vi "Solution part 2.vi"() -> ()   [LabVIEW 2020]
panel:
  out "Loop results":u64[](array[numeric])
  out "Total result":u64
  in  "data?":bool
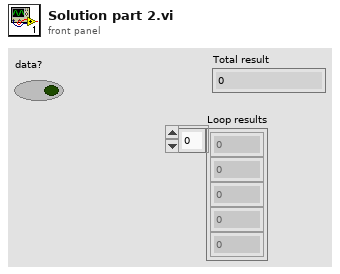
[diagram p1: front panel]
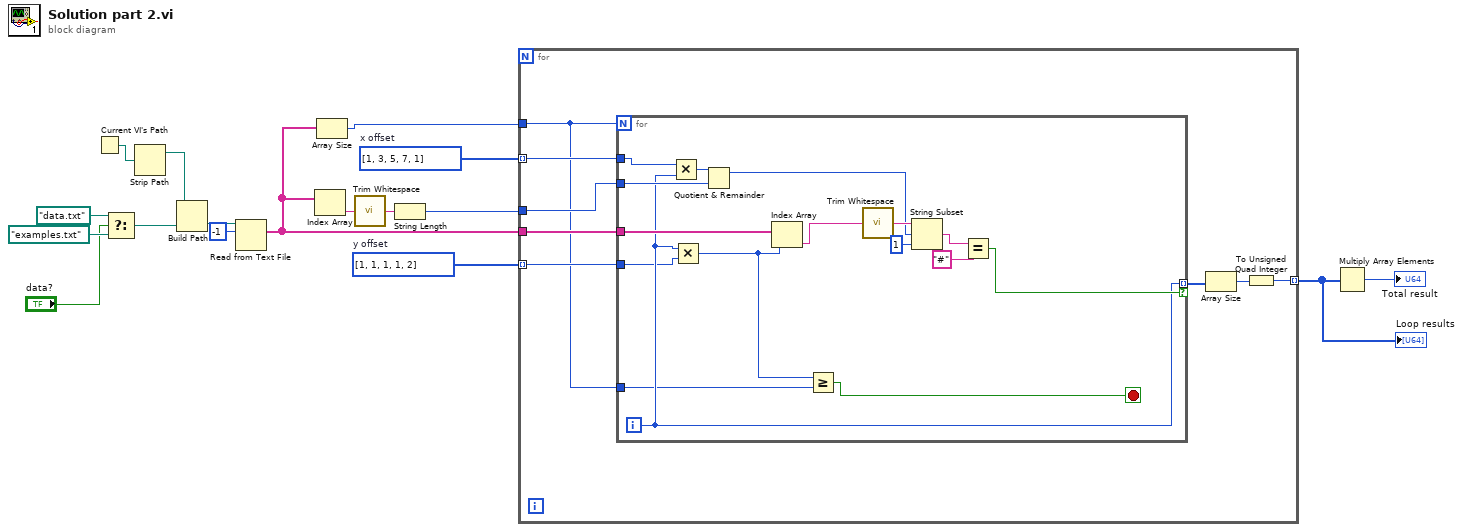
[diagram p0: block diagram]
diagram:
  w1 = i32[] [1, 3, 5, 7, 1]  # x offset
  w2 = i32[] [1, 1, 1, 1, 2]  # y offset
  n1 = Current VI's Path() -> (path=w13:path)
  n2 = Select(t=path "data.txt", s="data?", f=path "examples.txt") -> (s? t:f=w14:path)
  n3 = Strip Path(path=w13) -> (stripped path=w12:path)  [unwired: 1 out]
  n4 = Build Path(base path=w12, name or relative path=w14) -> (appended path=w11:path)
  n5 = Read from Text File(file (use dialog)=w11, count=-1) -> (text=w6:string[])  [unwired: 2 in, 3 out]
  n6 = Index Array(array=w6) -> (element=w9:string)  [unwired: 1 in]
  n7 = Array Size(array=w6) -> (size(s)=w5:i32)
  n8 = call <vilib>:"Trim Whitespace.vi"("string"=w9) -> ("trimmed string"=w7:string)  [unwired: 1 in]
  n9 = String Length(string=w7) -> (length=w8:i32)
  n10 = for {
    tunnel: [w18] -> w4 mode=indexing
    tunnel: w8 -> [w23]
    tunnel: w6 -> [w22]
    tunnel: w5 -> [w19]
    tunnel: w2 -> [w21] mode=indexing
    tunnel: w1 -> [w20] mode=indexing
    n11 = for {
      N: w19 -> [_]
      tunnel: w22 -> [w32]
      tunnel: [w31] -> w25 mode=indexing if=w37
      tunnel: w23 -> [w41]
      tunnel: w20 -> [w35]
      tunnel: w21 -> [w30]
      tunnel: w19 -> [w28]
      i -> [w31]
      stop <- w26 stop-if-true
      n12 = Multiply(x=w35, y=w31) -> (x*y=w34:i32)
      n13 = Multiply(x=w31, y=w30) -> (x*y=w27:i32)
      n14 = Quotient & Remainder(x=w34, y=w41) -> (x-y*floor(x/y)=w33:i32)  [unwired: 1 out]
      n15 = Index Array(array=w32, index=w27) -> (element=w29:string)
      n16 = Greater Or Equal?(x=w27, y=w28) -> (x >= y?=w26:bool)
      n17 = call <vilib>:"Trim Whitespace.vi"("string"=w29) -> ("trimmed string"=w36:string)  [unwired: 1 in]
      n18 = String Subset(string=w36, offset (0)=w33, length (rest)=1 ("length (rest)")) -> (substring=w39:string)
      n19 = Equal?(x=w39, y="#") -> (x = y?=w37:bool)
    }
    n20 = Array Size(array=w25) -> (size(s)=w24:i32)
    n21 = To Unsigned Quad Integer(1:w24) -> (0:w18:u64)
  }
  "Loop results" <- w4
  n22 = Multiply Array Elements(1:w4) -> (0:→"Total result":u64)
